vi "read.vi"(7 "timeout (ms)":i32, 8 "error in (no error)":errorcluster, 9 "number of channels":i32, 10 "block size":i32, 11 "FPGAWrapperMH120124RAPS_PXI7813R in":refnum<class "FPGAWrapperMH120124RAPS_PXI7813R.lvclass">) -> (0 "error out":errorcluster, 1 "channels raw data block":T1, 2 "FIFO full?":bool, 3 "FPGAWrapperMH120124RAPS_PXI7813R out":refnum<class "FPGAWrapperMH120124RAPS_PXI7813R.lvclass">, 4 "timed out?":bool)   [LabVIEW 2010, in "FPGAWrapperMH120124RAPS_PXI7813R.lvclass"]
uses:
  FPGAWrapperMH120124RAPS_PXI7813R.lvclass
  common/arrays/pixel_raw_data_array.ctl
  class_data.vi
  D:/Program Files/National Instruments/LabVIEW 2010/resource/objmgr/ni.dex.rc
panel:
  out "AvailElmntsForRead":i32
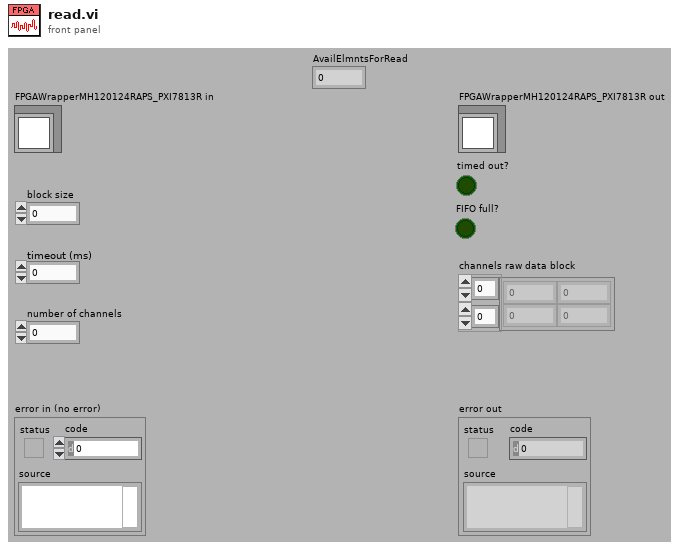
[diagram p1: front panel]
types:
  T1 = typedef "pixel_raw_data_array.ctl" = dbl[][]
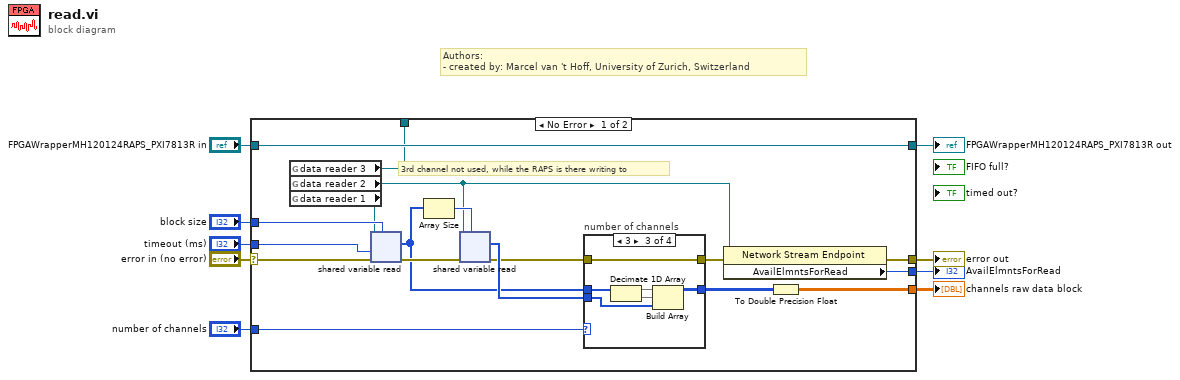
[diagram p0: block diagram]
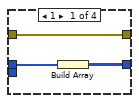
[diagram p2: hidden frame]
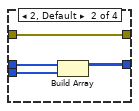
[diagram p3: hidden frame]
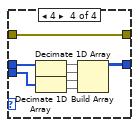
[diagram p4: hidden frame]
diagram:
  # "Authors: \n- created by: Marcel van 't Hoff, University of Zurich, Switzerland"
  n1 = case shown="No Error" "error in (no error)" {
    selector: "error in (no error)" -> [w26 w50]
    tunnel: [w18 w50] -> w7
    tunnel: [w27 w49] -> w8
    tunnel: "FPGAWrapperMH120124RAPS_PXI7813R in" -> [w27 w49]
    tunnel: "block size" -> [w25 _]
    tunnel: "timeout (ms)" -> [w24 _]
    tunnel: "number of channels" -> [w22 _]
    tunnel: [w20 _] -> w1
    tunnel: [w16 _] -> w2
    tunnel: [w10 _] -> _
    frame No Error {
      # "3rd channel not used, while the RAPS is there writing to"
      n2 = global read "class_data.vi" "data reader 3"() -> (w10:refnum<k21>)
      n3 = global read "class_data.vi" "data reader 2"() -> (w12:refnum<k21>)
      n4 = global read "class_data.vi" "data reader 1"() -> (w13:refnum<k21>)
      n5 = shared-variable-read(w13, w26, w24, w25) -> (w23:errorcluster, w15:u32[])  [unwired: 2 out]
      n6 = Array Size(array=w15) -> (size(s)=w14:i32)
      n7 = shared-variable-read(w12, w23, w14) -> (w11:errorcluster, w19:u32[])  [unwired: 1 in, 2 out]
      n8 = case "number of channels" shown="3" w22 {
        tunnel: w15 -> [w30 w34 w38 w46]
        tunnel: [w29 w33 w40 w48] -> w21
        tunnel: [w28 w32 w39 w47] -> w17
        tunnel: w11 -> [w28 w32 w39 w47]
        tunnel: w19 -> [_ w31 w35 w45]
        frame 1 {
          n9 = Build Array(w30) -> (w29:u32[][])
        }
        frame 2, Default {
          n10 = Build Array(w34, w31) -> (w33:u32[][])
        }
        frame 3 {
          n11 = Decimate 1D Array(w38) -> (w37:u32[], w36:u32[])
          n12 = Build Array(w37, w36, w35) -> (w40:u32[][])
        }
        frame 4 {
          n13 = Decimate 1D Array(w46) -> (w44:u32[], w43:u32[])
          n14 = Decimate 1D Array(w45) -> (w42:u32[], w41:u32[])
          n15 = Build Array(w44, w43, w42, w41) -> (w48:u32[][])
        }
      }
      n16 = property class="Network Stream Endpoint"(reference=w12, error in=w17) -> (error out=w18:errorcluster, "AvailElmntsForRead"=w16:i32)  [unwired: 1 out]
      n17 = To Double Precision Float(number=w21) -> (double precision float=w20:dbl[][])
    }
    frame Error {
    }
  }
  "error out" <- w7
  "FPGAWrapperMH120124RAPS_PXI7813R out" <- w8
  "channels raw data block" <- w1
  "AvailElmntsForRead" <- w2
